vi "start.vi"(8 "error in (no error)":errorcluster, 11 "niDAQmxDO in":refnum<class "niDAQmxDO.lvclass">) -> (0 "error out":errorcluster, 3 "niDAQmxDO out":refnum<class "niDAQmxDO.lvclass">)   [LabVIEW 2011, in "Hardware.lvlib" / "Channels.lvlib" / "niDAQmxDO.lvclass"]
uses:
  niDAQmxDO.lvclass
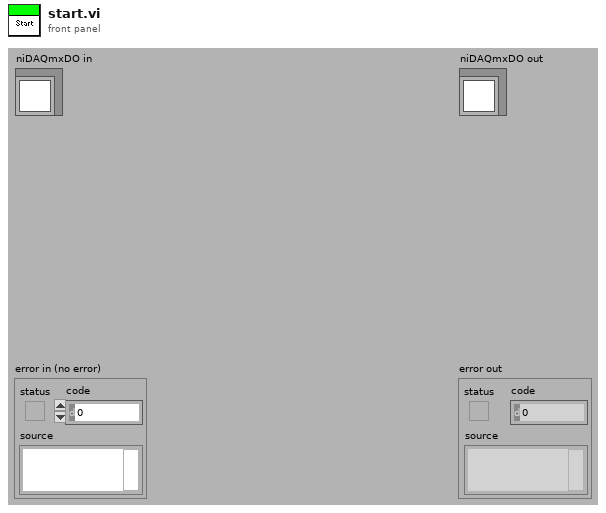
[diagram p1: front panel]
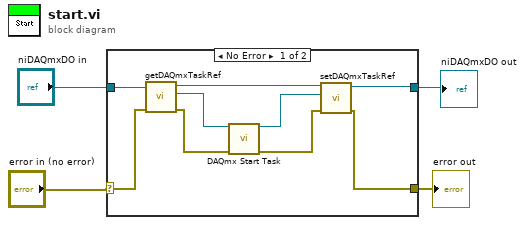
[diagram p0: block diagram]
diagram:
  n1 = case shown="No Error" "error in (no error)" {
    selector: "error in (no error)" -> [w12 w14]
    tunnel: "niDAQmxDO in" -> [w13 w15]
    tunnel: [w5 w15] -> w2
    tunnel: [w6 w14] -> w1
    frame No Error {
      n2 = call "getDAQmxTaskRef.vi"("error in (no error)"=w12, "niDAQmxDO.lvclass in"=w13) -> ("error out"=w10:errorcluster, "DAQmx Task Ref"=w11:refnum<k21>, "niDAQmxDO.lvclass out"=w9:refnum<class "niDAQmxDO.lvclass">)  [unwired: 7 in]
      n3 = call <vilib>:"DAQmx Start Task.vi"("task/channels in"=w11, "error in"=w10) -> ("task out"=w7:refnum<k21>, "error out"=w8:errorcluster)  [unwired: 12 in]
      n4 = call "setDAQmxTaskRef.vi"("error in (no error)"=w8, "DAQmx Task Ref"=w7, "niDAQmxDO.lvclass in"=w9) -> ("error out"=w6:errorcluster, "niDAQmxDO.lvclass out"=w5:refnum<class "niDAQmxDO.lvclass">)  [unwired: 7 in]
    }
    frame Error {
    }
  }
  "error out" <- w1
  "niDAQmxDO out" <- w2
